vi "initializeProgram.vi"(10 "subpanelRef":refnum<vi>, 11 "vi folder":path) -> ()   [LabVIEW 2015]
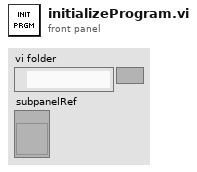
[diagram p1: front panel]
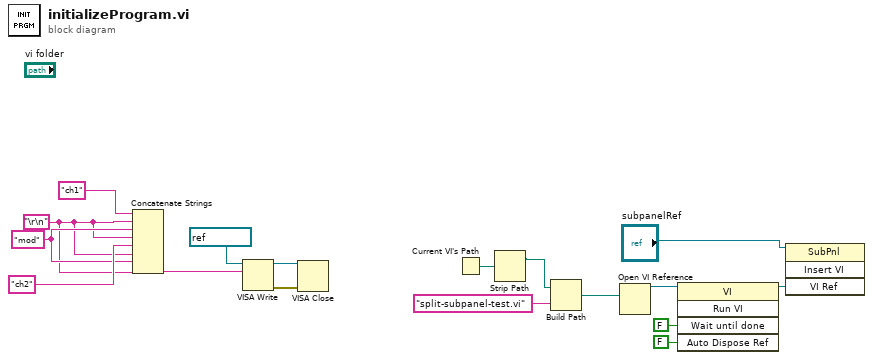
[diagram p0: block diagram]
diagram:
  w11 = "mod" ("f")
  w10 = "\r\n"
  n1 = Concatenate Strings("ch1" ("string"), w10, w11, w10, "ch2" ("string"), w10, w11, w10) -> (w14:string)
  n2 = VISA Write(VISA resource name=refnum<visa-resource-name> "COM3", write buffer=w14) -> (VISA resource name out=w8:refnum<visa-resource-name>, error out=w9:errorcluster)  [unwired: 1 in, 1 out]
  n3 = VISA Close(VISA resource name=w8, error in (no error)=w9) -> ()  [unwired: 1 out]
  n4 = Current VI's Path() -> (path=w16:path)
  n5 = Strip Path(path=w16) -> (stripped path=w2:path)  [unwired: 1 out]
  n6 = Build Path(base path=w2, name or relative path="split-subpanel-test.vi") -> (appended path=w17:path)
  n7 = Open VI Reference(vi path=w17) -> (vi reference=w4:refnum<vi>)  [unwired: 5 in, 1 out]
  n8 = invoke class="VI" method="Run VI"(reference=w4, "Wait until done"=FALSE ("Wait Until Done"), "Auto Dispose Ref"=FALSE ("Auto Dispose Reference")) -> (reference out=w3:refnum<vi>)  [unwired: 2 in, 4 out]
  n9 = invoke on="Invoke Node" class="SubPnl" method="Insert VI"(reference="subpanelRef", "VI Ref"=w3) -> ()  [unwired: 2 in, 4 out]
